vi "ChooseAuto.vi"   [LabVIEW 2014]
uses:
  <vilib>/Rock Robotics/Network Tables/SD Read Boolean.vi
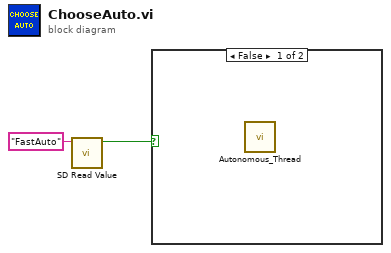
[diagram p0: block diagram]
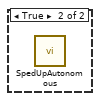
[diagram p2: hidden frame]
diagram:
  n1 = call-poly <vilib>:"SD Read Value.vi"("Name"="FastAuto") -> ("Boolean"=w2:bool)  [unwired: 8 in, 2 out]
  n2 = case shown="False" w2 {
    frame False {
      n3 = call "Autonomous_Thread.vi"() -> ()  [unwired: 1 in]
    }
    frame True {
      n4 = call "SpedUpAutonomous.vi"() -> ()  [unwired: 12 in]
    }
  }
